vi "mouse_ctrl get_down_pos.vi"(8 "error in (no error)":errorcluster, 11 "mouse_ctrl in":refnum<class "mouse_ctrl.lvclass">) -> (0 "error out":errorcluster, 2 "mouse down pos":cluster{"X":dbl, "Y":dbl}, 3 "mouse_ctrl out":refnum<class "mouse_ctrl.lvclass">)   [LabVIEW 2018, in "mouse_ctrl.lvclass"]
uses:
  mouse_ctrl.lvclass
  mouse_ctrl.lvclass/mouse_ctrl.ctl
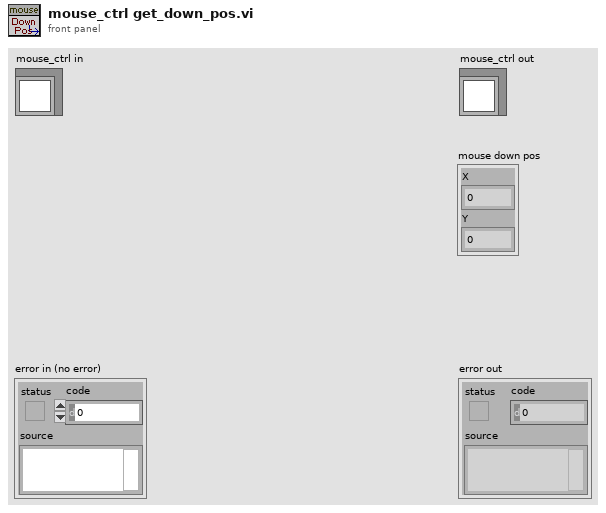
[diagram p1: front panel]
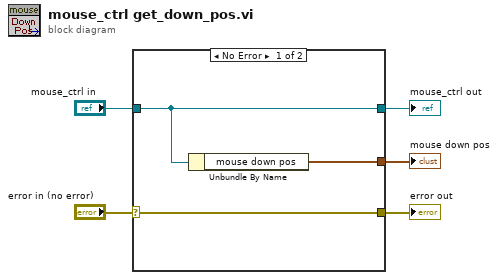
[diagram p0: block diagram]
diagram:
  n1 = case shown="No Error" "error in (no error)" {
    selector: "error in (no error)" -> [w8 w10]
    tunnel: [w8 w10] -> w4
    tunnel: [w7 w9] -> w2
    tunnel: "mouse_ctrl in" -> [w7 w9]
    tunnel: [w6 _] -> w1
    frame No Error {
      n2 = Unbundle By Name(w7) -> ("mouse down pos"=w6:cluster{"X":dbl, "Y":dbl})
    }
    frame Error {
    }
  }
  "error out" <- w4
  "mouse_ctrl out" <- w2
  "mouse down pos" <- w1
